vi "Measure.vi"(8 "error in (no error)":errorcluster, 9 "measurement configuration":variant, 10 "measure call context in":refnum<class "Measure Call Context.lvclass">, 11 "measurement plugin in":refnum<class "TDMS Waveform Creator.lvclass">) -> (0 "error out":errorcluster, 1 "measurement results":variant, 2 "measure call context out":refnum<class "Measure Call Context.lvclass">, 3 "measurement plugin out":refnum<class "TDMS Waveform Creator.lvclass">)   [LabVIEW 2025, in "TDMS Waveform Creator.lvclass"]
uses:
  TDMS Waveform Creator.lvclass
  TDMS Waveform Creator.lvclass/TDMS Waveform Creator.ctl
  Measurement Configuration.ctl
  <vilib>/Plug-In SDKs/Measurements/Measure Call Context/Measure Call Context.lvclass
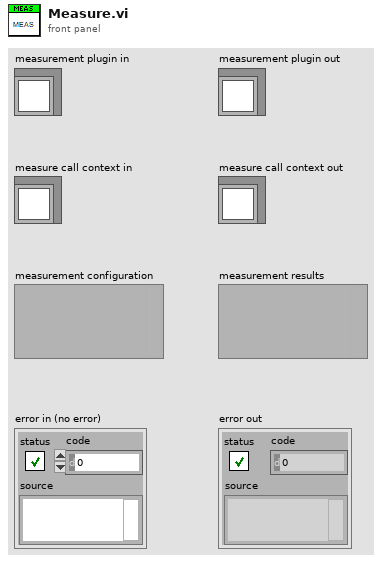
[diagram p1: front panel]
types:
  T1 = typedef "TDMS Waveform Creator.lvclass/Measurement Configuration.ctl" = cluster{"TDMS File Location":string, "Run Action":string, "Wfm Group Name":string, "Channel Names":string[], "Waveforms Summary JSON":string[]}
  T2 = typedef "TDMS Waveform Creator.lvclass/Measurement Results.ctl" = cluster{"Final Waveform Group Name":string}
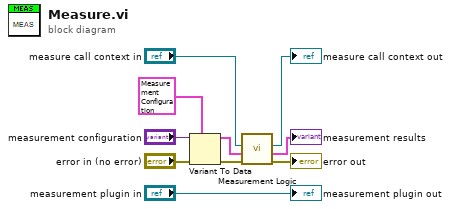
[diagram p0: block diagram]
diagram:
  n1 = Variant To Data(error in="error in (no error)", type=T1 {"TDMS File Location"="", "Run Action"="Lorem ipsum dolor sit", "Wfm Group Name"="Wfm1", "Channel Names"=[], "Waveforms Summary JSON"=[]} ("measurement configuration"), Variant="measurement configuration") -> (data=w1:T1, error out=w7:errorcluster)
  n2 = call "Measurement Logic.vi"("error in"=w7, "measurement configuration"=w1, "measure call context in"="measure call context in") -> ("error out"=→"error out":errorcluster, "measurement results"=→"measurement results":T2, "measure call context out"=→"measure call context out":refnum<class "Measure Call Context.lvclass">)  [unwired: 6 in]
  "measurement plugin out" <- "measurement plugin in"
